vi "kruispunt.vi"(10 "keuze 1,2 of 3":i32) -> ()   [LabVIEW 2019]
uses:
  <vilib>/myRIO/Common/Instrument Driver Framework/Utilities/typedefs/Analog Scaling Constants.ctl
  <vilib>/myRIO/Common/Instrument Driver Framework/Utilities/typedefs/Analog Scaling Constants List.ctl
  <vilib>/myRIO/Common/Instrument Driver Framework/myRIO v1.0/AO/typedefs/AO Channels Enum.ctl
  <vilib>/myRIO/Common/Instrument Driver Framework/myRIO v1.0/AO/typedefs/AO Channels List.ctl
  <vilib>/myRIO/Common/Instrument Driver Framework/Utilities/typedefs/Generic FPGA Reference.ctl
  <vilib>/myRIO/Common/Instrument Driver Framework/Utilities/typedefs/myRIO v1.0 Reference.ctl
  <vilib>/myRIO/Common/Instrument Driver Framework/Utilities/typedefs/Hardware Version Enum.ctl
  <vilib>/myRIO/Common/Instrument Driver Framework/Utilities/typedefs/myRIO Generic Hardware Reference.ctl
  <vilib>/myRIO/Instrument Drivers/Onboard IO/AO/typedefs/AO Reference.ctl
  <vilib>/myRIO/Instrument Drivers/Onboard IO/AO/AO.lvlib
  <vilib>/myRIO/Instrument Drivers/Onboard IO/AO/vis/Write.vi
  <vilib>/userDefined/High Color/nirio_resource_hc.ctl
  <vilib>/myRIO/Common/Instrument Driver Framework/myRIO v1.0/AO/vis/myRIO v1.1 Open AO.vi
  <vilib>/myRIO/Instrument Drivers/Onboard IO/AO/vis/myRIO AO Open.xnode
  <vilib>/myRIO/Common/Instrument Driver Framework/Utilities/vis/Is FPGA Ref Available.vi
  <vilib>/myRIO/Express VI/Onboard IO/AO/AO Express VI.xnode
  <vilib>/myRIO/Common/Instrument Driver Framework/myRIO v1.0/DIO/typedefs/DIO Channels Enum.ctl
  <vilib>/myRIO/Common/Instrument Driver Framework/myRIO v1.0/DIO/typedefs/DIO Channels List.ctl
  <vilib>/myRIO/Instrument Drivers/Onboard IO/DIO/typedefs/DIO Reference.ctl
  <vilib>/myRIO/Instrument Drivers/Onboard IO/DIO/DIO.lvlib
  <vilib>/myRIO/Instrument Drivers/Onboard IO/DIO/vis/Read.vi
  <vilib>/myRIO/Instrument Drivers/Onboard IO/DIO/vis/myRIO DIO Open.xnode
  <vilib>/myRIO/Express VI/Onboard IO/DI/DI Express VI.xnode
  <vilib>/myRIO/Instrument Drivers/Onboard IO/I2C/typedefs/I2C Transfer Rate.ctl
  <vilib>/myRIO/Instrument Drivers/Onboard IO/I2C/I2C.lvlib
  <vilib>/myRIO/Instrument Drivers/Onboard IO/I2C/typedefs/I2C User Configuration.ctl
  <vilib>/myRIO/Instrument Drivers/Onboard IO/I2C/typedefs/I2C Configuration.ctl
  <vilib>/myRIO/Common/Instrument Driver Framework/myRIO v1.0/I2C/typedefs/I2C Channels Enum.ctl
  <vilib>/myRIO/Instrument Drivers/Onboard IO/I2C/typedefs/I2C Reference.ctl
  <vilib>/myRIO/Instrument Drivers/Onboard IO/I2C/vis/Configure.vi
  <vilib>/myRIO/Instrument Drivers/Onboard IO/I2C/vis/Write.vi
  <vilib>/myRIO/Common/Instrument Driver Framework/myRIO v1.0/I2C/vis/myRIO v1.1 Open I2C.vi
  <vilib>/myRIO/Instrument Drivers/Onboard IO/I2C/vis/myRIO I2C Open.xnode
  <vilib>/myRIO/Express VI/Onboard IO/I2C/I2C Express VI.xnode
  interface.vi
  <vilib>/myRIO/Common/Instrument Driver Framework/myRIO v1.0/DIO/vis/myRIO v1.1 Open DIO.vi
panel:
  out "aantal significant verschillend":i32
  out "array controle op rood":i32[](array[numeric])
  in  "error in (no error) 4":errorcluster
  out "error out 4":errorcluster
types:
  T1 = typedef "AO.lvlib/AO Reference.ctl" = cluster{"myRIO Reference":T2, "AO Channel List":T6, "AO Scaling Constant List":T8}
  T2 = typedef "myRIO Generic Hardware Reference.ctl" = cluster{"myRIO Model":T3, "myRIO Hardware Reference":T4}
  T3 = typedef "Hardware Version Enum.ctl" = enum16{"Unknown", "myRIO-1900", "myRIO-1950", "roboRIO", "NI ELVIS RIO CM", "ELVIS III"}
  T4 = typedef "myRIO v1.0 Reference.ctl" = cluster{"Generic FPGA Reference":T5, "Allow multiple opens":bool}
  T5 = typedef "Generic FPGA Reference.ctl" = refnum<k20>
  T6 = typedef "AO Channels List.ctl" = T7[]
  T7 = typedef "AO Channels Enum.ctl" = enum16{"Not Connected", "AudioOut/Left", "AudioOut/Right", "C/AO0", "C/AO1", "A/AO0", "A/AO1", "B/AO0", "B/AO1"}
  T8 = typedef "Analog Scaling Constants List.ctl" = T9[]
  T9 = typedef "Analog Scaling Constants.ctl" = cluster{"LSB Weight (Volts)":dbl, "Offset (Volts)":dbl, "Signed?":bool}
  T10 = typedef "nirio_resource_hc.ctl" = tag
  T11 = typedef "I2C.lvlib/I2C Reference.ctl" = cluster{"myRIO Reference":T2, "I2C Channels Enum":T12, "I2C Configuration":T13}
  T12 = typedef "I2C Channels Enum.ctl" = enum16{"Not Connected", "A/I2C", "B/I2C", "I2C/I2C"}
  T13 = typedef "I2C.lvlib/I2C Configuration.ctl" = cluster{"I2C Transfer Rate":T14}
  T14 = typedef "I2C.lvlib/I2C Transfer Rate.ctl" = enum16{"Standard mode (100 kbps)", "Fast mode (400 kbps)"}
  T15 = typedef "I2C.lvlib/I2C User Configuration.ctl" = cluster{"I2C Transfer Rate":T14}
  T16 = typedef "DIO.lvlib/DIO Reference.ctl" = cluster{"myRIO Reference":T2, "DIO Channels List":T17}
  T17 = typedef "DIO Channels List.ctl" = T18[]
  T18 = typedef "DIO Channels Enum.ctl" = enum16{"Not Connected", "C/DIO0", "C/DIO1", "C/DIO2", "C/DIO3", "C/DIO4", "C/DIO5", "C/DIO6", "C/DIO7", "A/DIO0", "A/DIO1", "A/DIO2", "A/DIO3", "A/DIO4", "A/DIO5", "A/DIO6", "A/DIO7", "A/DIO8", "A/DIO9", "A/DIO10", "A/DIO11", "A/DIO12", "A/DIO13", "A/DIO14", "A/DIO15", "A/DIO16", "A/DIO17", "A/DIO18", "A/DIO19", "B/DIO0", "B/DIO1", "B/DIO2", "B/DIO3", "B/DIO4", "B/DIO5", "B/DIO6", "B/DIO7", "B/DIO8", "B/DIO9", "B/DIO10", "B/DIO11", "B/DIO12", "B/DIO13", "B/DIO14", "B/DIO15", "B/DIO16", "B/DIO17", "B/DIO18", "B/DIO19", "LED0", "LED1", "LED2", "LED3", "Button0", "DIO/DIO0", "DIO/DIO1", "DIO/DIO2", "DIO/DIO3", "DIO/DIO4", "DIO/DIO5", "DIO/DIO6", "DIO/DIO7", "DIO/DIO8", "DIO/DIO9", "SPI/CS0", "SPI/CS1", "SPI/CS2", "SPI/CS3", "LED RADIO (Green)", "LED RADIO (Red)", "LED COMM (Green)", "LED COMM (Red)", "LED MODE (Green)", "LED MODE (Red)"}
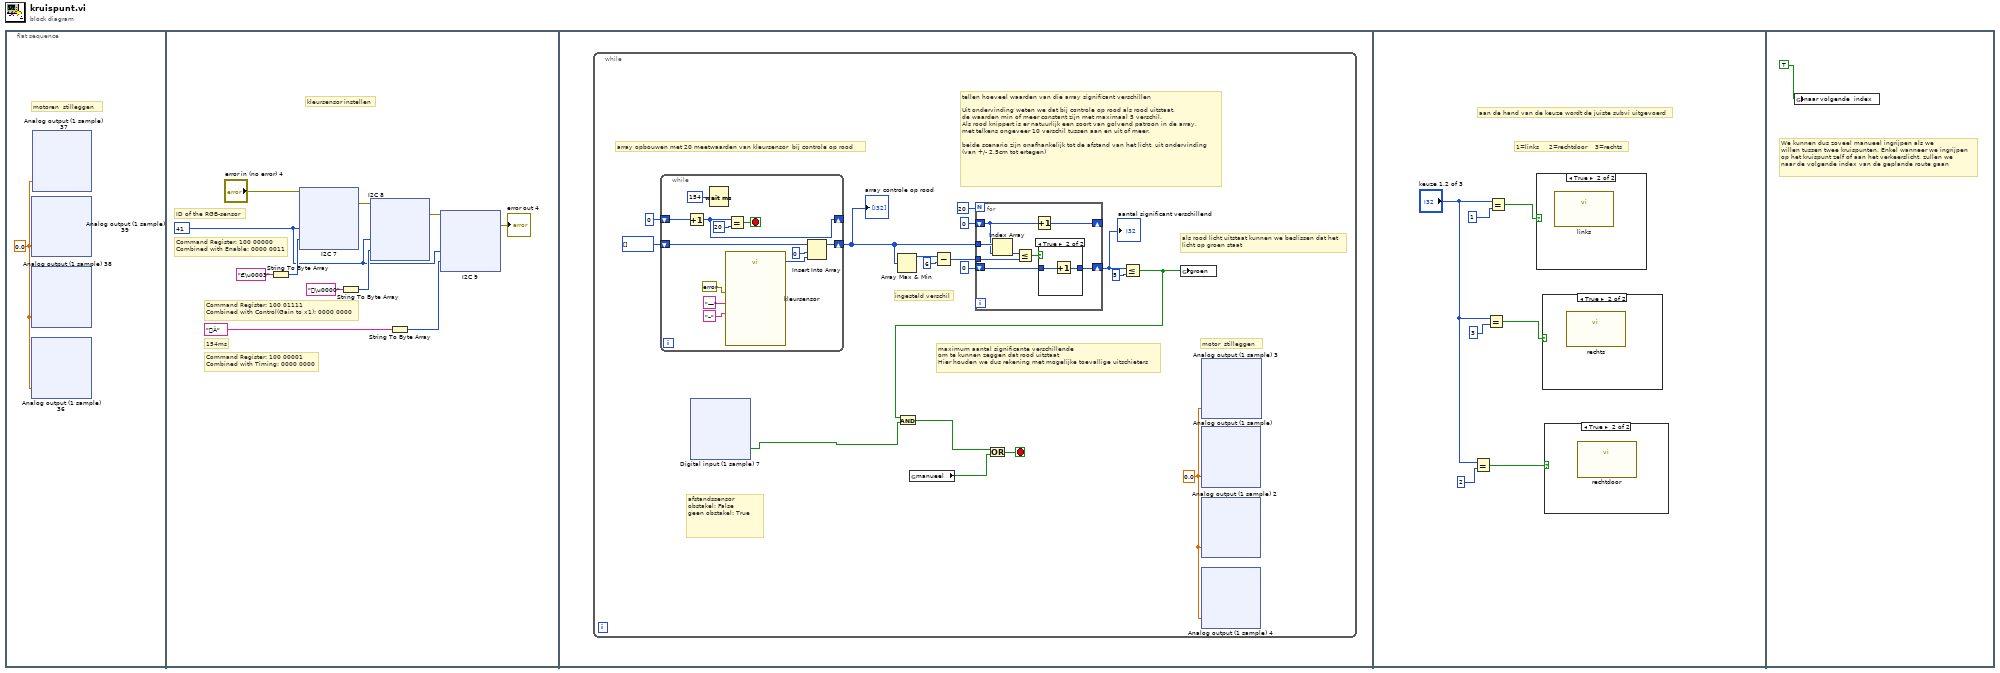
[diagram p0: block diagram]
diagram:
  n1 = flat-sequence {
    frame #0 {
      w1 = 0.0
      # "motoren  stilleggen"
      n2 = xnode "Analog output (1 sample) 39"("B/AO0 (Pin 2)"=w1) -> ()  [unwired: 1 in, 1 out]
      n3 = xnode "Analog output (1 sample) 38"("A/AO0 (Pin 2)"=w1) -> ()  [unwired: 1 in, 1 out]
      n4 = xnode "Analog output (1 sample) 36"("B/AO1 (Pin 4)"=w1) -> ()  [unwired: 1 in, 1 out]
      n5 = xnode "Analog output (1 sample) 37"("A/AO1 (Pin 4)"=w1) -> ()  [unwired: 1 in, 1 out]
    }
    frame #1 {
      w153 = 41 ("Numeric")
      # "kleursensor instellen"
      # "154ms"
      # "ID of the RGB-sensor"
      # "Command Register: 100 00000\nCombined with Enable: 0000 0011"
      # "Command Register: 100 01111\nCombined with Control(Gain to x1): 0000 0000"
      # "Command Register: 100 00001\nCombined with Timing: 0000 0000"
      n6 = String To Byte Array(string="€\u0003") -> (unsigned byte array=w154:u8[])
      n7 = xnode "I2C 7"("Slave Address (7-bit)"=w153, "Bytes to Write"=w154, "error in (no error)"="error in (no error) 4") -> ("error out"=w157:errorcluster)
      n8 = String To Byte Array(string="\u0000") -> (unsigned byte array=w155:u8[])
      n9 = xnode "I2C 8"("Slave Address (7-bit)"=w153, "Bytes to Write"=w155, "error in (no error)"=w157) -> ("error out"=w158:errorcluster)
      n10 = String To Byte Array(string="À") -> (unsigned byte array=w156:u8[])
      n11 = xnode "I2C 9"("Slave Address (7-bit)"=w153, "Bytes to Write"=w156, "error in (no error)"=w158) -> ("error out"=→"error out 4":errorcluster)
    }
    frame #2 {
      n12 = while {
        stop <- w290 stop-if-true
        w289 = 0.0
        # "als rood licht uitstaat kunnen we beslissen dat het\nlicht op groen staat"
        # "maximum aantal significante verschillende\nom te kunnen zeggen dat rood uitstaat\nHier houden we dus rekening met mogelijke toevallige uitschieters"
        # "ingesteld verschil"
        # "tellen hoeveel waarden van die array significant verschillen\n\nUit ondervinding weten we dat bij controle op rood als rood uitstaat,\nde waarden min of meer constant zijn met maximaal 5 verschil.\nAls rood knippert is er natuurlijk een soort van golvend patroon in de array,\nmet telkens ongeveer 10 verschil tussen aan en uit of meer.\n\nbeide scenario zijn onafhankelijk tot de afstand van het licht, uit ondervinding \n(van +/- 2,5cm tot ertegen)"
        # "array opbouwen met 20 meetwaarden van kleursensor  bij controle op rood"
        # "afstandssensor \nobstakel: False\ngeen obstakel: True"
        # "motor  stilleggen"
        n13 = while {
          shift-right: [w312] -> w275
          shift-left: i32[] [] -> [w311]
          shift-right: [w308] -> _
          shift-left: 0 -> [w310]
          stop <- w309 stop-if-true
          n14 = Increment(x=w310) -> (x+1=w308:i32)
          n15 = Wait (ms)(milliseconds to wait=u32 154) -> ()  [unwired: 1 out]
          n16 = call "kleursensor.vi"("error in (no error)"=errorcluster {"status"=FALSE, "code"=0, "source"=""}, "High 4"="—", "Low 4"="–") -> ("Total"=w303:u32)  [unwired: 5 in, 3 out]
          n17 = Equal?(x=w308, y=20) -> (x = y?=w309:bool)
          n18 = Insert Into Array(array=w311, index=0, new element=w303) -> (w312:i32[])
        }
        "array controle op rood" <- w275
        n19 = xnode "Digital input (1 sample) 7"() -> ("A/DIO1 (Pin 13)"=w287:bool)  [unwired: 1 in, 1 out]
        n20 = Array Max & Min(array=w275) -> (max value=w278:i32)  [unwired: 3 out]
        n21 = global read "interface.vi" "manueel"() -> (w291:bool)
        n22 = Subtract(x=w278, y=6) -> (x-y=w280:i32)
        n23 = for {
          N: 20 -> [_]
          tunnel: w275 -> [w299]
          shift-right: [w298] -> _
          shift-left: 0 -> [w297]
          tunnel: w280 -> [w294]
          shift-right: [w292] -> w277
          shift-left: 0 -> [w293]
          n24 = Index Array(array=w299, index=w297) -> (element=w295:i32)
          n25 = Less Or Equal?(x=w295, y=w294) -> (x <= y?=w296:bool)
          n26 = Increment(x=w297) -> (x+1=w298:i32)
          n27 = case shown="True" w296 {
            tunnel: w293 -> [w300 w302]
            tunnel: [w300 w301] -> w292
            frame False {
            }
            frame True {
              n28 = Increment(x=w302) -> (x+1=w301:i32)
            }
          }
        }
        "aantal significant verschillend" <- w277
        n29 = Less Or Equal?(x=w277, y=5) -> (x <= y?=w286:bool)
        n30 = And(x=w286, y=w287) -> (x .and. y?=w288:bool)
        n31 = Or(x=w288, y=w291) -> (x .or. y?=w290:bool)
        n32 = global write "interface.vi" "groen"(w286) -> ()
        n33 = xnode "Analog output (1 sample)"("B/AO0 (Pin 2)"=w289) -> ()  [unwired: 1 in, 1 out]
        n34 = xnode "Analog output (1 sample) 2"("A/AO0 (Pin 2)"=w289) -> ()  [unwired: 1 in, 1 out]
        n35 = xnode "Analog output (1 sample) 4"("B/AO1 (Pin 4)"=w289) -> ()  [unwired: 1 in, 1 out]
        n36 = xnode "Analog output (1 sample) 3"("A/AO1 (Pin 4)"=w289) -> ()  [unwired: 1 in, 1 out]
      }
    }
    frame #3 {
      # "aan de hand van de keuze wordt de juiste subvi uitgevoerd"
      # "1=links     2=rechtdoor    3=rechts"
      n37 = Equal?(x="keuze 1,2 of 3", y=2) -> (x = y?=w502:bool)
      n38 = Equal?(x="keuze 1,2 of 3", y=3) -> (x = y?=w503:bool)
      n39 = Equal?(x="keuze 1,2 of 3", y=1) -> (x = y?=w504:bool)
      n40 = case shown="True" w504 {
        frame False {
        }
        frame True {
          n41 = call "links.vi"() -> ()  [unwired: 12 in]
        }
      }
      n42 = case shown="True" w503 {
        frame False {
        }
        frame True {
          n43 = call "rechts.vi"() -> ()  [unwired: 12 in]
        }
      }
      n44 = case shown="True" w502 {
        frame False {
        }
        frame True {
          n45 = call "rechtdoor.vi"() -> ()  [unwired: 12 in]
        }
      }
    }
    frame #4 {
      # "We kunnen dus zoveel manueel ingrijpen als we\nwillen tussen twee kruispunten. Enkel wanneer we ingrijpen\nop het kruispunt zelf of aan het verkeerslicht, zullen we \nnaar de volgende index van de geplande route gaan"
      n46 = global write "interface.vi" "naar volgende  index"(TRUE) -> ()
    }
  }
